vi "Close.vi"(7 "path override":path, 8 "error in (no error)":errorcluster, 11 "s_":u64) -> (0 "error out":errorcluster)   [LabVIEW 2025, in "libzmq-v143-mt-4_3_6.lvlib"]
doc: "ZMQ_EXPORT int zmq_close (void *s_);"
uses:
  libzmq-v143-mt-4_3_6.lvlib
  errno.vi
  strerror.vi
  <vilib>/Utility/error.llb/Error Cluster From Error Code.vi
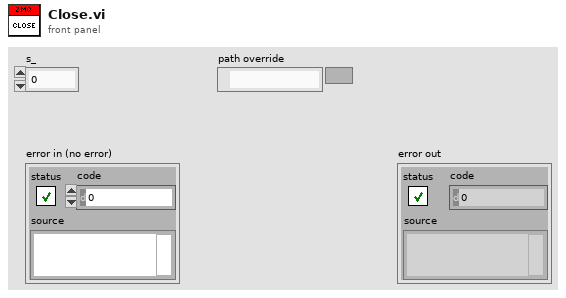
[diagram p1: front panel]
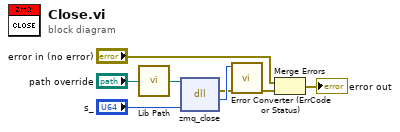
[diagram p0: block diagram]
diagram:
  n1 = call "Lib Path.vi"("path override"="path override") -> ("lib path"=w2:path)
  n2 = dll-call lib="home/james/Documents/ZeroMQ_LV/libzmq-v143-mt-4_3_6/libzmq.so" fn="zmq_close"(path in=w2, "s_"="s_") -> (error out=w1:errorcluster, "return type"=w8:i32)  [unwired: 3 in, 1 out]
  n3 = call "Error Converter (ErrCode or Status).vi"("error in (no error)"=w1, "error code"=w8) -> ("error out"=w6:errorcluster)  [unwired: 9 in]
  n4 = Merge Errors("error in (no error)", w6) -> (→"error out":errorcluster)
